vi "Raw Socket Ping.vi"(0 "Host to Ping":string="127.0.0.127", 1 "TTL":u8=128 min=1, 2 "Data Size in Bytes (32)":i32=32, 3 "Sequence Number":u16 format="%04x", 4 "Timeout (ms)":i32=1000) -> (5 "RxCount":i32 caption="Packets Received", 7 "Ping Reply Info":T1 {"Sequence" format="%04x"}, 9 "Timed Out?":bool)   [LabVIEW 2018]
uses:
  Ping Reply Info.ctl
panel:
  out "RxBytes":i32 caption="Bytes\nReceived\nBack"
  out "Socket Out":u32 caption="Socket ID Obtained" format="%04x"
  out "Resolved Host IP":u32 format="%x"
  out "Error Out":errorcluster
  in  "Error In":errorcluster
  out "Bytes Sent":i32
  # "Raw Socket Ping\nAdapted from http://tangentsoft.net/wskfaq/examples/rawping.html"
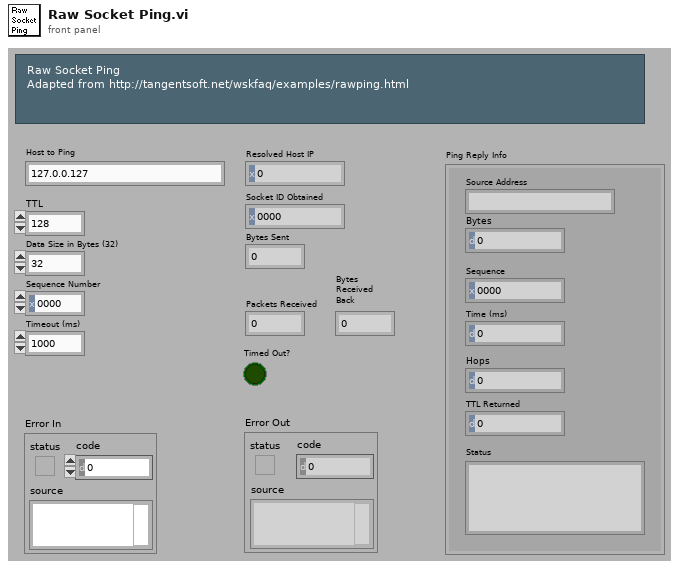
[diagram p1: front panel]
types:
  T1 = typedef "Ping Reply Info.ctl" = cluster{"Source Address":string, "Bytes":i32, "Sequence":u16, "Time (ms)":i32, "Hops":u8, "TTL Returned":u8, "Status":string}
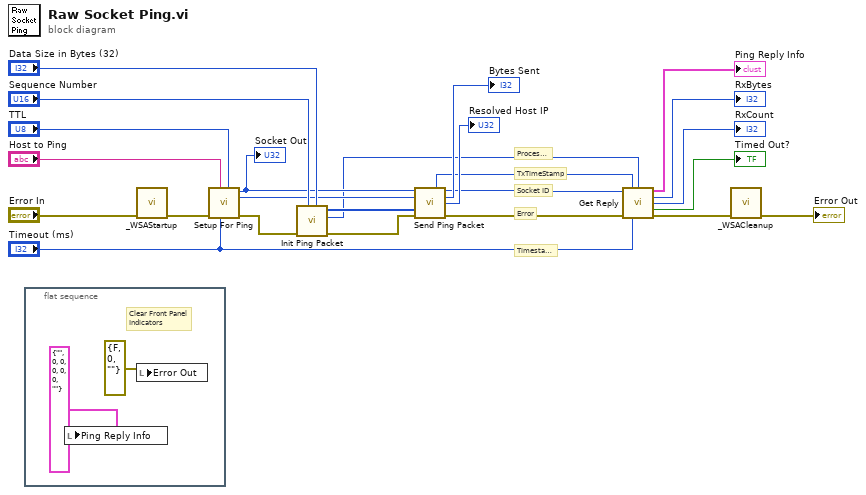
[diagram p0: block diagram]
diagram:
  # "Error"
  # "Timestamp"
  # "TxTimeStamp"
  # "Socket ID"
  # "ProcessID"
  n1 = flat-sequence {
    frame #0 {
      # "Clear Front Panel\nIndicators"
      n2 = local write "Ping Reply Info"(T1 {"Source Address"="", "Bytes"=0, "Sequence"=0, "Time (ms)"=0, "Hops"=0, "TTL Returned"=0, "Status"=""} ("Ping Reply Info")) -> ()
      n3 = local write "Error Out"(errorcluster {"status"=FALSE, "code"=0, "source"=""} ("Error Out")) -> ()
    }
  }
  n4 = call "_WSAStartup.vi"("Error In"="Error In") -> ("Error out"=w24:errorcluster)  [unwired: 9 in, 1 out]
  n5 = call "Setup For Ping.vi"("TTL (U8)"="TTL", "Timeout (ms)"="Timeout (ms)", "Host to Ping"="Host to Ping", "Error In"=w24) -> ("Error Out"=w22:errorcluster, "Resolved IP"=w13:u32, "Socket Out"=w12:u32)  [unwired: 5 in]
  "Socket Out" <- w12
  n6 = call "Init Ping Packet.vi"("Data Size in Bytes (32)"="Data Size in Bytes (32)", "Sequence Number"="Sequence Number", "Error In"=w22) -> ("Error Out"=w21:errorcluster, "ProcessID"=w6:u32, "Output Packet"=w11:u8[])  [unwired: 6 in]
  n7 = call "Send Ping Packet.vi"("Socket To Use"=w12, "Resolved Host IP"=w13, "Packet to Send"=w11, "Error In"=w21) -> ("TxTimeStamp"=w7:u32, "Socket To Use Out"=w10:u32, "Bytes Sent"=→"Bytes Sent":i32, "Resolved Host IP Out"=→"Resolved Host IP":u32, "Error Out"=w9:errorcluster)  [unwired: 7 in]
  n8 = call "Get Reply.vi"("Socket"=w10, "TxTimeStamp Alt"=w7, "ProcessID"=w6, "Error In"=w9, "Timeout (ms)"="Timeout (ms)") -> ("Ping Reply Info"=→"Ping Reply Info":T1, "RxBytes"=→"RxBytes":i32, "RxCount"=→"RxCount":i32, "Timed Out?"=→"Timed Out?":bool, "Error Out"=w5:errorcluster)  [unwired: 6 in]
  n9 = call "_WSACleanup.vi"("Error In"=w5) -> ("Error Out"=→"Error Out":errorcluster)  [unwired: 10 in]
